vi "Add Port.vi"(8 "error in":errorcluster, 9 "direction":T1, 10 "port number":u16, 11 "custom device ref":T2 format="%.0x") -> (0 "error out":errorcluster, 2 "port ref out":T2 format="%.0x", 3 "custom device ref out":T2 format="%.0x")   [LabVIEW 2020, in "ARINC 429 Scripting.lvlib"]
uses:
  ARINC 429 Scripting.lvlib
  <vilib>/NI VeriStand/Custom Device API/Custom Device Item Ref.ctl
  Shared/Direction.ctl
  Ballard/Constants.vi
  <vilib>/NI VeriStand/Custom Device Tools/Custom Device Utility Library/NI VeriStand - Search for Item by GUID.vi
  <vilib>/NI VeriStand/Custom Device API/Set Item Property (U16).vi
  <vilib>/NI VeriStand/Custom Device API/Custom Device API.lvlib
  Ballard/Ballard ARINC 429 Scripting.lvlib
  <vilib>/NI VeriStand/Custom Device Tools/Custom Device Utility Library/Custom Device Utility Library.lvlib
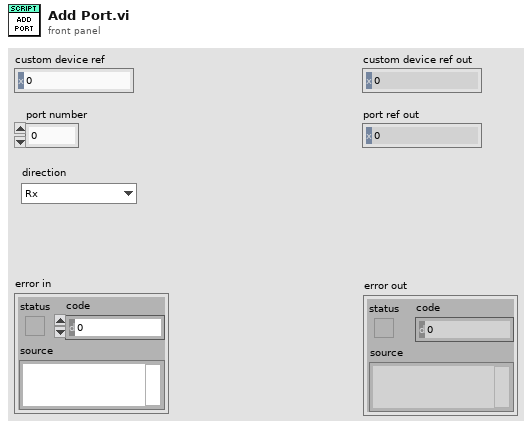
[diagram p1: front panel]
types:
  T1 = typedef "Direction.ctl" = enum16{"Rx", "Tx"}
  T2 = typedef "Custom Device API.lvlib/Custom Device Item Ref.ctl" = u64
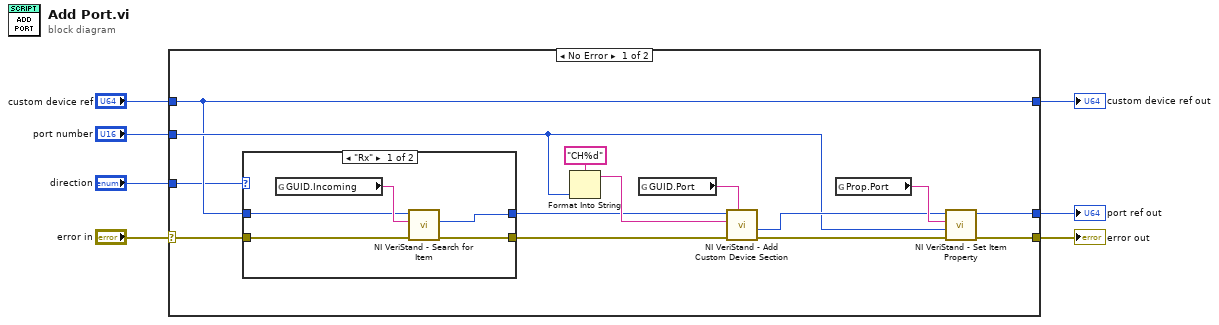
[diagram p0: block diagram]
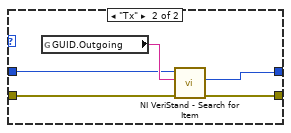
[diagram p2: hidden frame]
diagram:
  n1 = case shown="No Error" "error in" {
    selector: "error in" -> [w12 w33]
    tunnel: "custom device ref" -> [w9 w32]
    tunnel: [w18 w33] -> w6
    tunnel: [w16 _] -> w5
    tunnel: "port number" -> [w13 _]
    tunnel: [w9 w32] -> w2
    tunnel: "direction" -> [w8 _]
    frame No Error {
      n2 = case shown="\"Rx\"" w8 {
        tunnel: w9 -> [w23 w29]
        tunnel: [w24 w27] -> w10
        tunnel: w12 -> [w22 w30]
        tunnel: [w25 w28] -> w11
        frame "Rx" {
          n3 = global read "Constants.vi" "GUID.Incoming"() -> (w26:string)
          n4 = call-poly <vilib>:"NI VeriStand - Search for Item.vi"("error in"=w22, "Item GUID"=w26, "Section Ref in"=w23) -> ("error out"=w25:errorcluster, "Item Ref"=w24:T2)  [unwired: 5 in, 2 out]
        }
        frame "Tx" {
          n5 = global read "Constants.vi" "GUID.Outgoing"() -> (w31:string)
          n6 = call-poly <vilib>:"NI VeriStand - Search for Item.vi"("error in"=w30, "Item GUID"=w31, "Section Ref in"=w29) -> ("error out"=w28:errorcluster, "Item Ref"=w27:T2)  [unwired: 5 in, 2 out]
        }
      }
      n7 = Format Into String(format string="CH%d", w13) -> (resulting string=w14:string)  [unwired: 2 in, 1 out]
      n8 = global read "Constants.vi" "GUID.Port"() -> (w21:string)
      n9 = call <vilib>:"NI VeriStand - Add Custom Device Section.vi"("GUID (Default Section)"=w21, "error in (no error)"=w11, "Section Name"=w14, "Parent Ref in"=w10) -> ("error out"=w19:errorcluster, "Section Ptr"=w17:T2)  [unwired: 4 in, 2 out]
      n10 = global read "Constants.vi" "Prop.Port"() -> (w20:string)
      n11 = call-poly <vilib>:"NI VeriStand - Set Item Property.vi"("error in (no error)"=w19, "Value"=w13, "Property Name"=w20, "Item Ref in"=w17) -> ("error out"=w18:errorcluster, "Item Ref out"=w16:T2)  [unwired: 5 in, 1 out]
    }
    frame Error {
    }
  }
  "error out" <- w6
  "port ref out" <- w5
  "custom device ref out" <- w2
